vi "initializeILCOutputs.vi"(8 "error in (no error)":errorcluster, 11 "Model in":refnum<class "Model.lvclass">) -> (0 "error out":errorcluster, 3 "Model out":refnum<class "Model.lvclass">)   [LabVIEW 2016, in "Model.lvclass"]
uses:
  Model.lvclass
  Common_ILC/Typedefs/Outputs.ctl
  Model.lvclass/Model.ctl
  Common_ILC/ILC/ILC.lvclass/ILC.ctl
  Common_ILC/ILC/ILC.lvclass
  Common_ILC/Typedefs/ILCTypedefs.lvlib
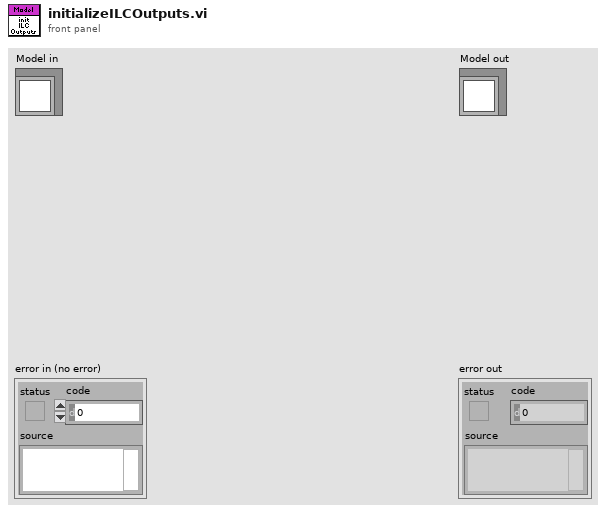
[diagram p1: front panel]
types:
  T1 = typedef "ILCCommon.lvlib/ILCTypedefs.lvlib/Outputs.ctl" = cluster{"Step & Direction":i16, "Blower RPM":u8, "PWM (SSR)":u8, "Ch1":u16, "Ch2":u16, "Ch3":u16, "Ch4":u16}
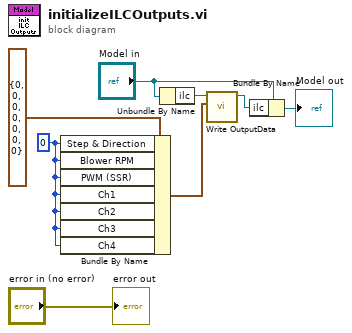
[diagram p0: block diagram]
diagram:
  w1 = i16 0 ("Step & Direction")
  n1 = Bundle By Name(cluster=T1 {"Step & Direction"=0, "Blower RPM"=0, "PWM (SSR)"=0, "Ch1"=0, "Ch2"=0, "Ch3"=0, "Ch4"=0} ("OutputData"), "Step & Direction"=w1, "Blower RPM"=w1, "PWM (SSR)"=w1, "Ch1"=w1, "Ch2"=w1, "Ch3"=w1, "Ch4"=w1) -> (w2:T1)
  n2 = Unbundle By Name("Model in") -> ("ilc"=w4:refnum<class "ILC.lvclass">)
  n3 = call "Write OutputData.vi"("OutputData"=w2, "ILC in"=w4) -> ("ILC out"=w5:refnum<class "ILC.lvclass">)  [unwired: 9 in]
  n4 = Bundle By Name(cluster="Model in", "ilc"=w5) -> (→"Model out":refnum<class "Model.lvclass">)
  "error out" <- "error in (no error)"
